vi "Lab Panel V6.00.vi"() -> ()   [LabVIEW 2017] (continued)
                n2898 = Index Array(array=w5298, index=4) -> (element=w5301:bool)
                n2899 = Not(x=w5301) -> (.not. x?=w5299:bool)
                n2900 = And(x=w5299, y=w5297) -> (x .and. y?=w5296:bool)
                n2901 = case shown="True" w5296 {
                  tunnel: w5304 -> [_ w5318]
                  tunnel: w5302 -> [_ w5315]
                  tunnel: w5303 -> [_ w5314]
                  frame False {
                  }
                  frame True {
                    n2902 = local read "TEMP START LAB05-2"() -> (w5320:cluster{"TL":dbl, "TN":dbl})
                    n2903 = local read "FAIL LAB05-2"() -> (w5311:cluster{"LO":dbl, "HI":dbl})
                    n2904 = local read "TDMS LAB05-2"() -> (w5319:refnum<k34>)
                    n2905 = local read "SET LAB05-2"() -> (w5316:T5)
                    n2906 = local read "DISP LAB05-2"() -> (w5317:T4)
                    n2907 = local read "SIG LAB05-2"() -> (w5321:T2)
                    n2908 = local read "RESULT LAB05-2"() -> (w5308:bool)
                    n2909 = Bundle("FAIL LAB05-2"=w5311, "SIG LAB05-2"=w5321, "TEMP START LAB05-2"=w5320, "DISP LAB05-2"=w5317, "SET LAB05-2"=w5316, "TDMS LAB05-2"=w5319) -> (w5306:T46)  [unwired: 1 in]
                    n2910 = call "sub vi - cycle&temp fail v7.vi"("Amps Lo?"=w5318, "Input Cluster"=w5306, "SELECT"=w5315, "Amps Hi?"=w5314, "Result In"=w5308, "Panel"=u64 10) -> ("(FAIL) out"=w5310:cluster{"FAIL LO":dbl, "FAIL HI":dbl}, "(DISP) out"=w5313:T4, "T-RISE"=w5307:cluster{"T-RISE (L)":dbl, "T-RISE (N)":dbl}, "Result Out"=w5309:bool, "file error"=w5312:errorcluster)  [unwired: 9 in]
                    n2911 = local write "TEMP RISE LAB05-2"(w5307) -> ()
                    n2912 = local write "FAIL LAB05-2"(w5310) -> ()
                    n2913 = local write "DISP LAB05-2"(w5313) -> ()
                    n2914 = local write "RESULT LAB05-2"(w5309) -> ()
                    n2915 = local write "data file error"(w5312) -> ()
                  }
                }
              }
            }
            n2916 = global write "Global 1.vi" "fail count"(w5035) -> ()
          }
          frame #17 {
            # "run calibration routine"
            n2917 = local read "SET (cal)"() -> (w5322:bool)
            n2918 = case shown="True" w5322 {
              frame False {
              }
              frame True {
                n2919 = stacked-sequence {
                  seq-local: [w5323 _ _] -> [_ w5325 _]
                  frame #0 {
                    n2920 = call "CALIBRATION PASSWORD"() -> ("PASSWORD"=w5323:string)  [unwired: 17 in, 2 out]
                  }
                  frame #1 {
                    n2921 = Equal?(x=w5325, y="7777") -> (x = y?=w5324:bool)
                    n2922 = case shown="True" w5324 {
                      frame False {
                      }
                      frame True {
                        n2923 = stacked-sequence {
                          frame #0 {
                            n2924 = local read "SAMPLES"() -> (w5327:dbl)
                            n2925 = local read "AI Task2"() -> (w5328:u32)
                            n2926 = local read "AI Task1"() -> (w5329:u32)
                            n2927 = local read "AI Task0"() -> (w5330:u64)
                            n2928 = local read "Temp Test Cal"() -> (w5331:dbl)
                            n2929 = call "sub vi - calibration v2.vi"("Samples"=w5327, "Task2"=w5328, "Task1"=w5329, "Task0"=w5330, "Temp Test Cal"=w5331) -> ()  [unwired: 7 in]
                          }
                          frame #1 {
                            n2930 = call "sub vi - get calibration values v1.vi"() -> ("TEMP REF CAL"=w5332:dbl, "LAB01 (CAL)"=w5337:T15, "LAB02 (CAL)"=w5336:T16, "LAB03 (CAL)"=w5335:T15, "LAB04 (CAL)"=w5334:T15, "calibration file error out"=w5338:errorcluster, "LAB05 (CAL)"=w5333:T15)  [unwired: 9 in]
                            n2931 = local write "TEMP REF cal"(w5332) -> ()
                            n2932 = local write "cal file error out"(w5338) -> ()
                            n2933 = local write "CAL LAB04"(w5334) -> ()
                            n2934 = local write "CAL LAB05"(w5333) -> ()
                            n2935 = local write "CAL LAB01"(w5337) -> ()
                            n2936 = local write "CAL LAB02"(w5336) -> ()
                            n2937 = local write "CAL LAB03"(w5335) -> ()
                          }
                        }
                      }
                    }
                  }
                  frame #2 {
                    n2938 = local write "SET (cal)"(FALSE) -> ()
                  }
                }
              }
            }
          }
          frame #18 {
            # "save certain settings to file"
            n2939 = String To Path(string="c:\\crabtree\\Set Up\\") -> (path=w5341:path)
            n2940 = Build Path(base path=w5341, name or relative path="settings.bin") -> (appended path=w5343:path)
            n2941 = Build Path(base path=w5341, name or relative path="mail.bin") -> (appended path=w5340:path)
            n2942 = Create Folder(path (use dialog)=w5341) -> (error out=w5346:errorcluster)  [unwired: 2 in, 2 out]
            n2943 = call <vilib>:"Clear Errors.vi"("error in (no error)"=w5346) -> ()  [unwired: 5 in, 2 out]
            n2944 = stacked-sequence {
              seq-local: [w5358 _] -> [_ w5371]
              tunnel: w5343 -> [_ w5372]
              tunnel: w5340 -> [_ w5370]
              frame #0 {
                n2945 = local read "C drive data root dir"() -> (w5357:path)
                n2946 = local read "Select COM port"() -> (w5354:refnum<visa-resource-name>)
                n2947 = local read "Network Directory"() -> (w5363:path)
                n2948 = local read "SET LAB05-2"() -> (w5362:T5)
                n2949 = local read "SET LAB05-1"() -> (w5361:T5)
                n2950 = local read "SET LAB04-2"() -> (w5360:T5)
                n2951 = local read "SET LAB03-2"() -> (w5364:T5)
                n2952 = local read "SET LAB04-1"() -> (w5359:T5)
                n2953 = local read "SET LAB03-1"() -> (w5365:T5)
                n2954 = local read "SET LAB02-2"() -> (w5366:T5)
                n2955 = local read "SET LAB02-1"() -> (w5367:T5)
                n2956 = local read "SET LAB01-2"() -> (w5368:T5)
                n2957 = local read "SET LAB01-1"() -> (w5369:T6)
                n2958 = local read "Temp Delay Lps"() -> (w5353:dbl)
                n2959 = local read "Amps Fail level"() -> (w5349:dbl)
                n2960 = local read "Temp Test Cal"() -> (w5350:dbl)
                n2961 = local read "Temp Value"() -> (w5352:dbl)
                n2962 = local read "Mail Test File To:"() -> (w5348:string)
                n2963 = local read "Fail Loops"() -> (w5351:dbl)
                n2964 = local read "Mail Test Fail"() -> (w5347:bool)
                n2965 = local read "RATE (Hz)"() -> (w5356:dbl)
                n2966 = local read "SAMPLES"() -> (w5355:dbl)
                n2967 = Bundle("SET LAB01-1"=w5369, "SET LAB01-2"=w5368, "SET LAB02-1"=w5367, "SET LAB02-2"=w5366, "SET LAB03-1"=w5365, "SET LAB03-2"=w5364, "SET LAB04-1"=w5359, "SET LAB04-2"=w5360, "SET LAB05-1"=w5361, "SET LAB05-2"=w5362, "Network Directory"=w5363, "C drive data root dir"=w5357, "RATE (Hz)"=w5356, "SAMPLES"=w5355, "Select COM port"=w5354, "Temp Delay Lps"=w5353, "Temp Value"=w5352, "Fail Loops"=w5351, "Temp Test Cal"=w5350, "Amps Fail level"=w5349, "Mail Test File To:"=w5348, "Mail Test Fail"=w5347) -> (w5358:T25)  [unwired: 1 in]
              }
              frame #1 {
                n2968 = event shown="[1] \"SET LAB01-1\", \"SET LAB01-2\", \"SET LAB02-1\", \"SET LAB02-2\", \"SET LAB03-1\", \"SET LAB03-2\", \"SET LAB04-1\", \"SET LAB04-2\", \"SET LAB05-1\", \"SET LAB05-2\", \"Network Directory\", \"C drive data root dir\", \"RATE (Hz)\", \"SAMPLES\", \"Select COM port\", \"Temp Delay Lps\", \"Temp Value\", \"Fail Loops\", \"Temp Test Cal\", \"Amps Fail level\", \"Mail Test File To:\", \"Mail Test Fail\": Value Change" {
                  selector: _ -> [_ _ _]
                  dyn-events: _ -> [_ _ _]
                  timeout: 10.0 -> [_ _ _]
                  tunnel: w5372 -> [_ w5374 _]
                  tunnel: w5371 -> [_ w5375 _]
                  tunnel: w5370 -> [_ _ w5386]
                  event Timeout {
                    n2969 = event-data() -> ()  [unwired: 1 in, 3 out]
                  }
                  event "SET LAB01-2", "SET LAB02-1", "SET LAB02-2", "SET LAB03-1", "SET LAB03-2", "SET LAB04-1", "SET LAB04-2", "SET LAB05-1", "SET LAB05-2", "Network Directory", "C drive data root dir", "RATE (Hz)", "SAMPLES", "Select COM port", "Temp Delay Lps", "Temp Value", "Fail Loops", "Temp Test Cal", "Amps Fail level", "Mail Test File To:", "Mail Test Fail": Value Change {
                    n2970 = event-data() -> ()  [unwired: 1 in, 6 out]
                    n2971 = Open/Create/Replace File(file path (use dialog)=w5374, operation (0:open)=T18."replace or create") -> (refnum out=w5380:refnum<file>, error out=w5379:errorcluster)  [unwired: 4 in, 1 out]
                    n2972 = Write to Binary File(file (use dialog)=w5380, data=w5375, error in=w5379) -> (refnum out=w5378:refnum<file>, error out=w5377:errorcluster)  [unwired: 3 in, 1 out]
                    n2973 = Close File(refnum=w5378, error in=w5377) -> (error out=w5376:errorcluster)  [unwired: 1 out]
                    n2974 = local write "data file error"(w5376) -> ()
                  }
                  event "MAIL SETTINGS.OUT SERVER ADDRESS", "MAIL SETTINGS.FROM ACCOUNT", "MAIL SETTINGS.USER NAME", "MAIL SETTINGS.PASSWORD", "Auto Mail Send", "TO (string):": Value Change {
                    n2975 = event-data() -> ()  [unwired: 1 in, 6 out]
                    n2976 = local read "Auto Mail Send"() -> (w5383:bool)
                    n2977 = local read "MAIL SETTINGS"() -> (w5385:T8)
                    n2978 = local read "TO (string):"() -> (w5382:string)
                    n2979 = Open/Create/Replace File(file path (use dialog)=w5386, operation (0:open)=T18."replace or create") -> (refnum out=w5391:refnum<file>, error out=w5390:errorcluster)  [unwired: 4 in, 1 out]
                    n2980 = Bundle("MAIL SETTINGS"=w5385, "Auto Mail Send"=w5383, "TO (string):"=w5382) -> (w5384:T47)  [unwired: 1 in]
                    n2981 = Write to Binary File(file (use dialog)=w5391, data=w5384, error in=w5390) -> (refnum out=w5389:refnum<file>, error out=w5388:errorcluster)  [unwired: 3 in, 1 out]
                    n2982 = Close File(refnum=w5389, error in=w5388) -> (error out=w5387:errorcluster)  [unwired: 1 out]
                    n2983 = local write "data file error"(w5387) -> ()
                  }
                }
              }
            }
          }
          frame #19 {
            # "mail control"
            n2984 = local read "MAIL SETTINGS"() -> (w5408:T8)
            n2985 = local read "Auto Mail Send"() -> (w5394:bool)
            n2986 = Unbundle By Name(w5408) -> ("OUT SERVER ADDRESS"=w5407:string, "FROM ACCOUNT"=w5406:string, "TEST MAIL"=w5405:bool)
            n2987 = stacked-sequence {
              tunnel: "TO (string):" -> [_ w5447]
              tunnel: w5408 -> [w5413 w5446]
              tunnel: w5407 -> [w5412 w5445]
              tunnel: w5406 -> [w5411 w5444]
              tunnel: w5405 -> [w5410 _]
              tunnel: w5394 -> [_ w5443]
              tunnel: w5404 -> [_ w5442]
              tunnel: w5403 -> [_ w5441]
              tunnel: w5402 -> [_ w5440]
              tunnel: w5401 -> [_ w5439]
              tunnel: w5400 -> [_ w5438]
              tunnel: w5399 -> [_ w5437]
              tunnel: w5398 -> [_ w5436]
              tunnel: w5397 -> [_ w5435]
              tunnel: w5396 -> [_ w5434]
              tunnel: w5395 -> [_ w5433]
              tunnel: "TO (string):" -> [w5409 _]
              frame #0 {
                # "mail test"
                n2988 = case shown="True" w5410 {
                  tunnel: w5413 -> [_ w5417]
                  tunnel: w5409 -> [_ w5416]
                  tunnel: w5412 -> [_ w5415]
                  tunnel: w5411 -> [_ w5414]
                  frame False {
                  }
                  frame True {
                    n2989 = stacked-sequence {
                      seq-local: [_ _ w5427 _] -> [_ _ _ w5428]
                      tunnel: w5417 -> [w5420 _ _ w5432]
                      tunnel: w5416 -> [_ _ w5425 _]
                      tunnel: w5415 -> [_ _ w5423 _]
                      tunnel: w5414 -> [_ _ w5424 _]
                      frame #0 {
                        n2990 = Bundle(cluster=w5420, "TEST MAIL STATUS"="TEST START") -> (w5418:T8)  [unwired: 6 in]
                        n2991 = local write "MAIL SETTINGS"(w5418) -> ()
                      }
                      frame #1 {
                        n2992 = Wait (ms)(milliseconds to wait=500) -> ()  [unwired: 1 out]
                      }
                      frame #2 {
                        n2993 = call "Lab Send Mail Test.vi"("TO:"=w5425, "subject"="MAIL TEST FROM LAB PANEL", "from"=w5424, "out going server"=w5423, "message"="TEST MESSAGE") -> ("error out"=w5427:errorcluster)  [unwired: 10 in]
                      }
                      frame #3 {
                        n2994 = Bundle(cluster=w5432, "TEST MAIL"=FALSE, "TEST MAIL STATUS"="TEST END", "mail error"=w5428) -> (w5430:T8)  [unwired: 4 in]
                        n2995 = local write "MAIL SETTINGS"(w5430) -> ()
                      }
                    }
                  }
                }
              }
              frame #1 {
                # "mail report"
                n2996 = stacked-sequence {
                  seq-local: [_ w5490 _ _] -> [_ _ _ w5680]
                  seq-local: [_ _ w5593 _] -> [_ _ _ w5670]
                  seq-local: [w5457 _ _ _] -> [_ w5507 _ _]
                  seq-local: [w5456 _ _ _] -> [_ w5506 _ _]
                  seq-local: [w5454 _ _ _] -> [_ w5504 _ _]
                  seq-local: [w5455 _ _ _] -> [_ w5505 _ _]
                  seq-local: [w5453 _ _ _] -> [_ w5503 _ _]
                  seq-local: [w5452 _ _ _] -> [_ w5498 _ _]
                  seq-local: [w5451 _ _ _] -> [_ w5499 _ _]
                  seq-local: [w5450 _ _ _] -> [_ w5500 _ _]
                  seq-local: [w5449 _ _ _] -> [_ w5501 _ _]
                  seq-local: [w5448 _ _ _] -> [_ w5502 _ _]
                  tunnel: w5447 -> [_ _ _ w5681]
                  tunnel: w5446 -> [_ _ _ w5664]
                  tunnel: w5445 -> [_ _ _ w5678]
                  tunnel: w5444 -> [_ _ _ w5677]
                  tunnel: w5443 -> [w5488 _ _ w5672]
                  tunnel: w5442 -> [_ _ w5623 _]
                  tunnel: w5441 -> [_ _ w5620 _]
                  tunnel: w5440 -> [_ _ w5619 _]
                  tunnel: w5439 -> [_ _ w5618 _]
                  tunnel: w5438 -> [_ _ w5617 _]
                  tunnel: w5437 -> [_ _ w5616 _]
                  tunnel: w5436 -> [_ _ w5615 _]
                  tunnel: w5435 -> [_ _ w5614 _]
                  tunnel: w5434 -> [_ _ w5613 _]
                  tunnel: w5433 -> [_ _ w5612 _]
                  frame #0 {
                    n2997 = case shown="False" w5488 {
                      frame False {
                        n2998 = local write "mail control"("") -> ()
                      }
                      frame True {
                      }
                    }
                    n2999 = local read "SET LAB01-1"() -> (w5487:T6)
                    n3000 = local read "SET LAB01-2"() -> (w5486:T5)
                    n3001 = local read "SET LAB02-1"() -> (w5485:T5)
                    n3002 = local read "SET LAB02-2"() -> (w5484:T5)
                    n3003 = local read "SET LAB03-1"() -> (w5483:T5)
                    n3004 = local read "SET LAB04-1"() -> (w5481:T5)
                    n3005 = local read "SET LAB05-1"() -> (w5479:T5)
                    n3006 = local read "SET LAB03-2"() -> (w5482:T5)
                    n3007 = local read "SET LAB04-2"() -> (w5480:T5)
                    n3008 = local read "SET LAB05-2"() -> (w5478:T5)
                    n3009 = Unbundle(w5483) -> ("DESCRIPTION"=w5463:string)  [unwired: 4 out]
                    n3010 = Unbundle(w5482) -> ("DESCRIPTION"=w5462:string)  [unwired: 4 out]
                    n3011 = Unbundle(w5481) -> ("DESCRIPTION"=w5461:string)  [unwired: 4 out]
                    n3012 = Unbundle(w5478) -> ("DESCRIPTION"=w5458:string)  [unwired: 4 out]
                    n3013 = Unbundle(w5484) -> ("DESCRIPTION"=w5464:string)  [unwired: 4 out]
                    n3014 = Unbundle(w5480) -> ("DESCRIPTION"=w5460:string)  [unwired: 4 out]
                    n3015 = Unbundle(w5487) -> ("DESCRIPTION"=w5476:string)  [unwired: 4 out]
                    n3016 = Unbundle(w5485) -> ("DESCRIPTION"=w5465:string)  [unwired: 4 out]
                    n3017 = Unbundle(w5479) -> ("DESCRIPTION"=w5459:string)  [unwired: 4 out]
                    n3018 = Unbundle(w5486) -> ("DESCRIPTION"=w5466:string)  [unwired: 4 out]
                    n3019 = Concatenate Strings("[LAB05-2/", w5458) -> (w5448:string)
                    n3020 = Concatenate Strings("[LAB05-1/", w5459) -> (w5449:string)
                    n3021 = Concatenate Strings("[LAB04-2/", w5460) -> (w5450:string)
                    n3022 = Concatenate Strings("[LAB03-2/", w5462) -> (w5452:string)
                    n3023 = Concatenate Strings("[LAB04-1/", w5461) -> (w5451:string)
                    n3024 = Concatenate Strings("[LAB03-1/", w5463) -> (w5453:string)
                    n3025 = Concatenate Strings("[LAB01-2/", w5466) -> (w5456:string)
                    n3026 = Concatenate Strings("[LAB02-2/", w5464) -> (w5454:string)
                    n3027 = Concatenate Strings("[LAB01-1/", w5476) -> (w5457:string)
                    n3028 = Concatenate Strings("[LAB02-1/", w5465) -> (w5455:string)
                  }
                  frame #1 {
                    w5511 = "/"
                    w5512 = 2.0
                    n3029 = local read "DISP LAB01-1"() -> (w5592:T4)
                    n3030 = local read "DISP LAB01-2"() -> (w5591:T4)
                    n3031 = local read "DISP LAB02-1"() -> (w5590:T4)
                    n3032 = local read "DISP LAB03-2"() -> (w5587:T4)
                    n3033 = local read "DISP LAB02-2"() -> (w5589:T4)
                    n3034 = local read "DISP LAB03-1"() -> (w5588:T4)
                    n3035 = local read "DISP LAB04-2"() -> (w5585:T4)
                    n3036 = local read "DISP LAB04-1"() -> (w5586:T4)
                    n3037 = local read "DISP LAB05-1"() -> (w5584:T4)
                    n3038 = local read "DISP LAB05-2"() -> (w5583:T4)
                    n3039 = Unbundle By Name(w5592) -> ("CYCLE"=w5580:dbl, "MINS"=w5579:dbl, "STATUS"=w5576:string)
                    n3040 = Unbundle(w5591) -> ("CYCLE"=w5575:dbl, "MINS"=w5574:dbl, "STATUS"=w5571:string)
                    n3041 = Unbundle(w5590) -> ("CYCLE"=w5568:dbl, "MINS"=w5567:dbl, "STATUS"=w5566:string)
                    n3042 = Unbundle(w5587) -> ("CYCLE"=w5555:dbl, "MINS"=w5554:dbl, "STATUS"=w5551:string)
                    n3043 = Unbundle(w5588) -> ("CYCLE"=w5560:dbl, "MINS"=w5559:dbl, "STATUS"=w5556:string)
                    n3044 = Unbundle(w5589) -> ("CYCLE"=w5565:dbl, "MINS"=w5564:dbl, "STATUS"=w5561:string)
                    n3045 = Unbundle(w5586) -> ("CYCLE"=w5550:dbl, "MINS"=w5549:dbl, "STATUS"=w5546:string)
                    n3046 = Unbundle(w5585) -> ("CYCLE"=w5545:dbl, "MINS"=w5544:dbl, "STATUS"=w5541:string)
                    n3047 = Unbundle(w5584) -> ("CYCLE"=w5540:dbl, "MINS"=w5539:dbl, "STATUS"=w5536:string)
                    n3048 = Unbundle(w5583) -> ("CYCLE"=w5582:dbl, "MINS"=w5581:dbl, "STATUS"=w5533:string)
                    n3049 = Number To Decimal String(number=w5568) -> (decimal integer string=w5570:string)  [unwired: 1 in]
                    n3050 = Number To Decimal String(number=w5565) -> (decimal integer string=w5563:string)  [unwired: 1 in]
                    n3051 = Number To Decimal String(number=w5560) -> (decimal integer string=w5558:string)  [unwired: 1 in]
                    n3052 = Number To Decimal String(number=w5575) -> (decimal integer string=w5573:string)  [unwired: 1 in]
                    n3053 = Number To Decimal String(number=w5555) -> (decimal integer string=w5553:string)  [unwired: 1 in]
                    n3054 = Number To Decimal String(number=w5580) -> (decimal integer string=w5578:string)  [unwired: 1 in]
                    n3055 = Number To Decimal String(number=w5582) -> (decimal integer string=w5535:string)  [unwired: 1 in]
                    n3056 = Number To Decimal String(number=w5550) -> (decimal integer string=w5548:string)  [unwired: 1 in]
                    n3057 = Number To Decimal String(number=w5545) -> (decimal integer string=w5543:string)  [unwired: 1 in]
                    n3058 = Number To Decimal String(number=w5540) -> (decimal integer string=w5538:string)  [unwired: 1 in]
                    n3059 = Number To Fractional String(number=w5567, precision (6)=w5512) -> (F-format string=w5569:string)  [unwired: 2 in]
                    n3060 = Number To Fractional String(number=w5554, precision (6)=w5512) -> (F-format string=w5552:string)  [unwired: 2 in]
                    n3061 = Number To Fractional String(number=w5564, precision (6)=w5512) -> (F-format string=w5562:string)  [unwired: 2 in]
                    n3062 = Number To Fractional String(number=w5559, precision (6)=w5512) -> (F-format string=w5557:string)  [unwired: 2 in]
                    n3063 = Number To Fractional String(number=w5544, precision (6)=w5512) -> (F-format string=w5542:string)  [unwired: 2 in]
                    n3064 = Number To Fractional String(number=w5549, precision (6)=w5512) -> (F-format string=w5547:string)  [unwired: 2 in]
                    n3065 = Number To Fractional String(number=w5574, precision (6)=w5512) -> (F-format string=w5572:string)  [unwired: 2 in]
                    n3066 = Number To Fractional String(number=w5539, precision (6)=w5512) -> (F-format string=w5537:string)  [unwired: 2 in]
                    n3067 = Number To Fractional String(number=w5579, precision (6)=w5512) -> (F-format string=w5577:string)  [unwired: 2 in]
                    n3068 = Number To Fractional String(number=w5581, precision (6)=w5512) -> (F-format string=w5534:string)  [unwired: 2 in]
                    n3069 = Concatenate Strings(w5511, w5553, w5511, w5552, w5511, w5551) -> (w5527:string)
                    n3070 = Concatenate Strings(w5511, w5548, w5511, w5547, w5511, w5546) -> (w5526:string)
                    n3071 = Concatenate Strings(w5511, w5543, w5511, w5542, w5511, w5541) -> (w5525:string)
                    n3072 = Concatenate Strings(w5511, w5538, w5511, w5537, w5511, w5536) -> (w5524:string)
                    n3073 = Concatenate Strings(w5511, w5535, w5511, w5534, w5511, w5533) -> (w5523:string)
                    n3074 = Concatenate Strings(w5511, w5578, w5511, w5577, w5511, w5576) -> (w5532:string)
                    n3075 = Concatenate Strings(w5511, w5558, w5511, w5557, w5511, w5556) -> (w5528:string)
                    n3076 = Concatenate Strings(w5511, w5573, w5511, w5572, w5511, w5571) -> (w5531:string)
                    n3077 = Concatenate Strings(w5511, w5570, w5511, w5569, w5511, w5566) -> (w5530:string)
                    n3078 = Concatenate Strings(w5511, w5563, w5511, w5562, w5511, w5561) -> (w5529:string)
                    n3079 = Concatenate Strings("]", "\r") -> (w5508:string)
                    n3080 = Concatenate Strings(w5503, w5528, w5508) -> (w5518:string)
                    n3081 = Concatenate Strings(w5505, w5530, w5508) -> (w5520:string)
                    n3082 = Concatenate Strings(w5504, w5529, w5508) -> (w5519:string)
                    n3083 = Concatenate Strings(w5500, w5525, w5508) -> (w5515:string)
                    n3084 = Concatenate Strings(w5501, w5524, w5508) -> (w5516:string)
                    n3085 = Concatenate Strings(w5499, w5526, w5508) -> (w5514:string)
                    n3086 = Concatenate Strings(w5498, w5527, w5508) -> (w5513:string)
                    n3087 = Concatenate Strings(w5502, w5523, w5508) -> (w5517:string)
                    n3088 = Concatenate Strings(w5506, w5531, w5508) -> (w5521:string)
                    n3089 = Concatenate Strings(w5507, w5532, w5508) -> (w5522:string)
                    n3090 = Concatenate Strings(w5522, w5521, w5520, w5519, w5518, w5513, w5514, w5515, w5516, w5517) -> (w5491:string)
                    n3091 = Concatenate Strings("[PANEL/", "DESC/", "CYCLES/", "MINS/", "STATUS]", "\r", w5491) -> (w5490:string)
                    "MAIL REPORT" <- w5490
                    n3092 = global write "Global display 3.vi" "log all"(w5490) -> ()
                  }
                  frame #2 {
                    w5621 = "END"
                    n3093 = local read "mail control"() -> (w5622:string)
                    n3094 = case shown="False" w5617 {
                      tunnel: w5622 -> [w5646 _]
                      tunnel: w5621 -> [w5645 _]
                      tunnel: [w5644 FALSE] -> w5607
                      frame False {
                        n3095 = Equal?(x=w5646, y=w5645) -> (x = y?=w5644:bool)
                      }
                      frame True {
                      }
                    }
                    n3096 = case shown="False" w5623 {
                      tunnel: w5622 -> [w5662 _]
                      tunnel: w5621 -> [w5661 _]
                      tunnel: [w5660 FALSE] -> w5611
                      frame False {
                        n3097 = Equal?(x=w5662, y=w5661) -> (x = y?=w5660:bool)
                      }
                      frame True {
                      }
                    }
                    n3098 = case shown="False" w5620 {
                      tunnel: w5622 -> [w5658 _]
                      tunnel: w5621 -> [w5657 _]
                      tunnel: [w5656 FALSE] -> w5610
                      frame False {
                        n3099 = Equal?(x=w5658, y=w5657) -> (x = y?=w5656:bool)
                      }
                      frame True {
                      }
                    }
                    n3100 = case shown="False" w5618 {
                      tunnel: w5622 -> [w5650 _]
                      tunnel: w5621 -> [w5649 _]
                      tunnel: [w5648 FALSE] -> w5608
                      frame False {
                        n3101 = Equal?(x=w5650, y=w5649) -> (x = y?=w5648:bool)
                      }
                      frame True {
                      }
                    }
                    n3102 = case shown="False" w5619 {
                      tunnel: w5622 -> [w5654 _]
                      tunnel: w5621 -> [w5653 _]
                      tunnel: [w5652 FALSE] -> w5609
                      frame False {
                        n3103 = Equal?(x=w5654, y=w5653) -> (x = y?=w5652:bool)
                      }
                      frame True {
                      }
                    }
                    n3104 = Or(x=w5609, y=w5608) -> (x .or. y?=w5600:bool)
                    n3105 = Or(x=w5611, y=w5610) -> (x .or. y?=w5601:bool)
                    n3106 = Or(x=w5601, y=w5600) -> (x .or. y?=w5596:bool)
                    n3107 = case shown="False" w5613 {
                      tunnel: w5622 -> [w5630 _]
                      tunnel: w5621 -> [w5629 _]
                      tunnel: [w5628 FALSE] -> w5602
                      frame False {
                        n3108 = Equal?(x=w5630, y=w5629) -> (x = y?=w5628:bool)
                      }
                      frame True {
                      }
                    }
                    n3109 = case shown="False" w5612 {
                      tunnel: w5622 -> [w5626 _]
                      tunnel: w5621 -> [w5625 _]
                      tunnel: [w5624 FALSE] -> w5606
                      frame False {
                        n3110 = Equal?(x=w5626, y=w5625) -> (x = y?=w5624:bool)
                      }
                      frame True {
                      }
                    }
                    n3111 = case shown="False" w5614 {
                      tunnel: w5622 -> [w5634 _]
                      tunnel: w5621 -> [w5633 _]
                      tunnel: [w5632 FALSE] -> w5603
                      frame False {
                        n3112 = Equal?(x=w5634, y=w5633) -> (x = y?=w5632:bool)
                      }
                      frame True {
                      }
                    }
                    n3113 = case shown="False" w5616 {
                      tunnel: w5622 -> [w5642 _]
                      tunnel: w5621 -> [w5641 _]
                      tunnel: [w5640 FALSE] -> w5605
                      frame False {
                        n3114 = Equal?(x=w5642, y=w5641) -> (x = y?=w5640:bool)
                      }
                      frame True {
                      }
                    }
                    n3115 = case shown="False" w5615 {
                      tunnel: w5622 -> [w5638 _]
                      tunnel: w5621 -> [w5637 _]
                      tunnel: [w5636 FALSE] -> w5604
                      frame False {
                        n3116 = Equal?(x=w5638, y=w5637) -> (x = y?=w5636:bool)
                      }
                      frame True {
                      }
                    }
                    n3117 = Or(x=w5605, y=w5604) -> (x .or. y?=w5599:bool)
                    n3118 = Or(x=w5603, y=w5602) -> (x .or. y?=w5598:bool)
                    n3119 = Or(x=w5606, y=w5607) -> (x .or. y?=w5594:bool)
                    n3120 = Or(x=w5599, y=w5598) -> (x .or. y?=w5597:bool)
                    n3121 = Or(x=w5596, y=w5597) -> (x .or. y?=w5595:bool)
                    n3122 = Or(x=w5595, y=w5594) -> (x .or. y?=w5593:bool)
                  }
                  frame #3 {
                    n3123 = local read "on loops"() -> (w5676:dbl)
                    n3124 = local read "jig cycle"() -> (w5673:dbl)
                    n3125 = local read "Send Mail Now"() -> (w5667:bool)
                    n3126 = Add(x=w5676, y=5.0) -> (x+y=w5674:dbl)
                    n3127 = Equal?(x=w5673, y=w5674) -> (x = y?=w5668:bool)
                    n3128 = And(x=w5668, y=w5667) -> (x .and. y?=w5666:bool)
                    n3129 = And(x=w5672, y=w5668) -> (x .and. y?=w5671:bool)
                    n3130 = And(x=w5671, y=w5670) -> (x .and. y?=w5669:bool)
                    n3131 = Or(x=w5669, y=w5666) -> (x .or. y?=w5665:bool)
                    n3132 = case shown="True" w5665 {
                      tunnel: w5681 -> [_ w5687]
                      tunnel: w5680 -> [_ w5686]
                      tunnel: "Lab Panel Test Status" -> [_ w5685]
                      tunnel: w5678 -> [_ w5684]
                      tunnel: w5677 -> [_ w5683]
                      tunnel: w5664 -> [_ w5682]
                      frame False {
                      }
                      frame True {
                        n3133 = stacked-sequence {
                          tunnel: w5687 -> [w5696 _]
                          tunnel: w5686 -> [w5695 _]
                          tunnel: w5685 -> [w5694 _]
                          tunnel: w5684 -> [w5693 _]
                          tunnel: w5683 -> [w5692 _]
                          tunnel: w5682 -> [w5691 _]
                          frame #0 {
                            n3134 = call "Lab Send Mail Test.vi"("TO:"=w5696, "subject"=w5694, "Info"="Test station status report", "from"=w5692, "out going server"=w5693, "message"=w5695) -> ("error out"=w5690:errorcluster)  [unwired: 9 in]
                            n3135 = Bundle(cluster=w5691, "mail error"=w5690) -> (w5689:T8)  [unwired: 6 in]
                            n3136 = local write "MAIL SETTINGS"(w5689) -> ()
                          }
                          frame #1 {
                            n3137 = local write "mail control"("") -> ()
                            n3138 = local write "Send Mail Now"(FALSE) -> ()
                          }
                        }
                      }
                    }
                  }
                }
              }
            }
          }
          frame #20 {
            # "save jig cycle values once all run switches are off"
            n3139 = stacked-sequence {
              tunnel: w5708 -> [_ w5737]
              tunnel: w5707 -> [_ w5736]
              tunnel: w5706 -> [_ w5735]
              tunnel: w5705 -> [_ w5734]
              tunnel: w5704 -> [_ w5733]
              tunnel: w5703 -> [_ w5732]
              tunnel: w5702 -> [_ w5731]
              tunnel: w5701 -> [_ w5730]
              tunnel: w5700 -> [_ w5729]
              tunnel: w5699 -> [_ w5728]
              frame #0 {
              }
              frame #1 {
                n3140 = Not(x=w5728) -> (.not. x?=w5711:bool)
                n3141 = Not(x=w5736) -> (.not. x?=w5726:bool)
                n3142 = Not(x=w5733) -> (.not. x?=w5721:bool)
                n3143 = Not(x=w5731) -> (.not. x?=w5717:bool)
                n3144 = Not(x=w5729) -> (.not. x?=w5713:bool)
                n3145 = Not(x=w5737) -> (.not. x?=w5727:bool)
                n3146 = Not(x=w5735) -> (.not. x?=w5725:bool)
                n3147 = Not(x=w5732) -> (.not. x?=w5719:bool)
                n3148 = Not(x=w5734) -> (.not. x?=w5723:bool)
                n3149 = Not(x=w5730) -> (.not. x?=w5715:bool)
                n3150 = local read "Save JC"() -> (w5739:bool)
                n3151 = And(x=w5727, y=w5726) -> (x .and. y?=w5724:bool)
                n3152 = And(x=w5724, y=w5725) -> (x .and. y?=w5722:bool)
                n3153 = And(x=w5722, y=w5723) -> (x .and. y?=w5720:bool)
                n3154 = And(x=w5720, y=w5721) -> (x .and. y?=w5718:bool)
                n3155 = And(x=w5718, y=w5719) -> (x .and. y?=w5716:bool)
                n3156 = And(x=w5716, y=w5717) -> (x .and. y?=w5714:bool)
                n3157 = And(x=w5714, y=w5715) -> (x .and. y?=w5712:bool)
                n3158 = And(x=w5712, y=w5713) -> (x .and. y?=w5710:bool)
                n3159 = And(x=w5710, y=w5711) -> (x .and. y?=w5709:bool)
                n3160 = And(x=w5709, y=w5739) -> (x .and. y?=w5738:bool)
                n3161 = case shown="True" w5738 {
                  tunnel: w5709 -> [w5740 _]
                  frame False {
                    n3162 = case shown="False" w5740 {
                      frame False {
                        n3163 = local write "Save JC"(TRUE) -> ()
                      }
                      frame True {
                      }
                    }
                  }
                  frame True {
                    n3164 = stacked-sequence {
                      frame #0 {
                        n3165 = String To Path(string="c:\\crabtree\\Jig Cycles\\") -> (path=w5752:path)
                        n3166 = Build Path(base path=w5752, name or relative path="jigcycles.bin") -> (appended path=w5750:path)
                        n3167 = Create Folder(path (use dialog)=w5752) -> (error out=w5754:errorcluster)  [unwired: 2 in, 2 out]
                        n3168 = local read "JIG RELAY CYCLES"() -> (w5744:T9)
                        n3169 = call <vilib>:"Clear Errors.vi"("error in (no error)"=w5754) -> ()  [unwired: 5 in, 2 out]
                        n3170 = local write "Save JC"(FALSE) -> ()
                        n3171 = Open/Create/Replace File(file path (use dialog)=w5750, operation (0:open)=T18."replace or create") -> (refnum out=w5748:refnum<file>, error out=w5749:errorcluster)  [unwired: 4 in, 1 out]
                        n3172 = Write to Binary File(file (use dialog)=w5748, data=w5744, error in=w5749) -> (refnum out=w5747:refnum<file>, error out=w5746:errorcluster)  [unwired: 3 in, 1 out]
                        n3173 = Close File(refnum=w5747, error in=w5746) -> (error out=w5745:errorcluster)  [unwired: 1 out]
                        n3174 = local write "data file error"(w5745) -> ()
                      }
                      frame #1 {
                        n3175 = local read "JIG RELAY CYCLES"() -> (w5777:T9)
                        n3176 = Unbundle By Name(w5777) -> ("LAB01-1"=w5772:dbl, "LAB01-2"=w5771:dbl, "LAB02-1"=w5769:dbl, "LAB02-2"=w5768:dbl, "LAB03-1"=w5766:dbl, "LAB03-2"=w5763:dbl, "LAB04-1"=w5762:dbl, "LAB04-2"=w5760:dbl, "LAB05-1"=w5758:dbl, "LAB05-2"=w5756:dbl)
                        n3177 = stacked-sequence {
                          tunnel: w5772 -> [w5780 _ _ _ _ _ _ _ _ _]
                          tunnel: 1000000 -> [w5783 w5793 w5803 w5813 w5823 w5833 w5843 w5853 w5863 w5873]
                          tunnel: [w5781 _ _ _ _ _ _ _ _ _] -> w5775
                          tunnel: "TEST STATION HAS REACHED 1 MILLION CYCLES, REPLACE  CONTROL RELAYS" -> [w5779 w5791 w5801 w5811 w5821 w5831 w5841 w5851 w5861 w5871]
                          tunnel: [_ w5790 _ _ _ _ _ _ _ _] -> w5773
                          tunnel: w5771 -> [_ w5789 _ _ _ _ _ _ _ _]
                          tunnel: [_ _ w5800 _ _ _ _ _ _ _] -> w5770
                          tunnel: w5769 -> [_ _ w5799 _ _ _ _ _ _ _]
                          tunnel: w5768 -> [_ _ _ w5810 _ _ _ _ _ _]
                          tunnel: [_ _ _ w5809 _ _ _ _ _ _] -> w5767
                          tunnel: w5766 -> [_ _ _ _ w5820 _ _ _ _ _]
                          tunnel: [_ _ _ _ w5819 _ _ _ _ _] -> w5765
                          tunnel: [_ _ _ _ _ w5830 _ _ _ _] -> w5764
                          tunnel: w5763 -> [_ _ _ _ _ w5829 _ _ _ _]
                          tunnel: w5762 -> [_ _ _ _ _ _ w5840 _ _ _]
                          tunnel: [_ _ _ _ _ _ w5839 _ _ _] -> w5761
                          tunnel: w5760 -> [_ _ _ _ _ _ _ w5850 _ _]
                          tunnel: [_ _ _ _ _ _ _ w5849 _ _] -> w5759
                          tunnel: w5758 -> [_ _ _ _ _ _ _ _ w5860 _]
                          tunnel: [_ _ _ _ _ _ _ _ w5859 _] -> w5757
                          tunnel: w5756 -> [_ _ _ _ _ _ _ _ _ w5870]
                          tunnel: [_ _ _ _ _ _ _ _ _ w5869] -> w5755
                          frame #0 {
                            n3178 = Greater?(x=w5780, y=w5783) -> (0:w5782:bool)
                            n3179 = case shown="True" w5782 {
                              tunnel: [w5784 0] -> w5781
                              tunnel: w5780 -> [w5784 _]
                              tunnel: w5779 -> [_ w5785]
                              frame False {
                              }
                              frame True {
                                n3180 = Concatenate Strings("LA01-1 ", w5785) -> (w5788:string)
                                n3181 = One Button Dialog(message=w5788) -> ()  [unwired: 1 in, 1 out]
                              }
                            }
                          }
                          frame #1 {
                            n3182 = Greater?(x=w5789, y=w5793) -> (0:w5792:bool)
                            n3183 = case shown="True" w5792 {
                              tunnel: [w5794 0] -> w5790
                              tunnel: w5789 -> [w5794 _]
                              tunnel: w5791 -> [_ w5795]
                              frame False {
                              }
                              frame True {
                                n3184 = Concatenate Strings("LA01-2 ", w5795) -> (w5798:string)
                                n3185 = One Button Dialog(message=w5798) -> ()  [unwired: 1 in, 1 out]
                              }
                            }
                          }
                          frame #2 {
                            n3186 = Greater?(x=w5799, y=w5803) -> (0:w5802:bool)
                            n3187 = case shown="True" w5802 {
                              tunnel: [w5804 0] -> w5800
                              tunnel: w5799 -> [w5804 _]
                              tunnel: w5801 -> [_ w5805]
                              frame False {
                              }
                              frame True {
                                n3188 = Concatenate Strings("LA02-1 ", w5805) -> (w5808:string)
                                n3189 = One Button Dialog(message=w5808) -> ()  [unwired: 1 in, 1 out]
                              }
                            }
                          }
                          frame #3 {
                            n3190 = Greater?(x=w5810, y=w5813) -> (0:w5812:bool)
                            n3191 = case shown="True" w5812 {
                              tunnel: [w5814 0] -> w5809
                              tunnel: w5810 -> [w5814 _]
                              tunnel: w5811 -> [_ w5815]
                              frame False {
                              }
                              frame True {
                                n3192 = Concatenate Strings("LA02-2 ", w5815) -> (w5818:string)
                                n3193 = One Button Dialog(message=w5818) -> ()  [unwired: 1 in, 1 out]
                              }
                            }
                          }
                          frame #4 {
                            n3194 = Greater?(x=w5820, y=w5823) -> (0:w5822:bool)
                            n3195 = case shown="True" w5822 {
                              tunnel: [w5824 0] -> w5819
                              tunnel: w5820 -> [w5824 _]
                              tunnel: w5821 -> [_ w5825]
                              frame False {
                              }
                              frame True {
                                n3196 = Concatenate Strings("LA03-1 ", w5825) -> (w5828:string)
                                n3197 = One Button Dialog(message=w5828) -> ()  [unwired: 1 in, 1 out]
                              }
                            }
                          }
                          frame #5 {
                            n3198 = Greater?(x=w5829, y=w5833) -> (0:w5832:bool)
                            n3199 = case shown="True" w5832 {
                              tunnel: [w5834 0] -> w5830
                              tunnel: w5829 -> [w5834 _]
                              tunnel: w5831 -> [_ w5835]
                              frame False {
                              }
                              frame True {
                                n3200 = Concatenate Strings("LA03-2 ", w5835) -> (w5838:string)
                                n3201 = One Button Dialog(message=w5838) -> ()  [unwired: 1 in, 1 out]
                              }
                            }
                          }
                          frame #6 {
                            n3202 = Greater?(x=w5840, y=w5843) -> (0:w5842:bool)
                            n3203 = case shown="True" w5842 {
                              tunnel: [w5844 0] -> w5839
                              tunnel: w5840 -> [w5844 _]
                              tunnel: w5841 -> [_ w5845]
                              frame False {
                              }
                              frame True {
                                n3204 = Concatenate Strings("LA04-1 ", w5845) -> (w5848:string)
                                n3205 = One Button Dialog(message=w5848) -> ()  [unwired: 1 in, 1 out]
                              }
                            }
                          }
                          frame #7 {
                            n3206 = Greater?(x=w5850, y=w5853) -> (0:w5852:bool)
                            n3207 = case shown="True" w5852 {
                              tunnel: [w5854 0] -> w5849
                              tunnel: w5850 -> [w5854 _]
                              tunnel: w5851 -> [_ w5855]
                              frame False {
                              }
                              frame True {
                                n3208 = Concatenate Strings("LA04-2 ", w5855) -> (w5858:string)
                                n3209 = One Button Dialog(message=w5858) -> ()  [unwired: 1 in, 1 out]
                              }
                            }
                          }
                          frame #8 {
                            n3210 = Greater?(x=w5860, y=w5863) -> (0:w5862:bool)
                            n3211 = case shown="True" w5862 {
                              tunnel: [w5864 0] -> w5859
                              tunnel: w5860 -> [w5864 _]
                              tunnel: w5861 -> [_ w5865]
                              frame False {
                              }
                              frame True {
                                n3212 = Concatenate Strings("LA05-1 ", w5865) -> (w5868:string)
                                n3213 = One Button Dialog(message=w5868) -> ()  [unwired: 1 in, 1 out]
                              }
                            }
                          }
                          frame #9 {
                            n3214 = Greater?(x=w5870, y=w5873) -> (0:w5872:bool)
                            n3215 = case shown="True" w5872 {
                              tunnel: [w5874 0] -> w5869
                              tunnel: w5870 -> [w5874 _]
                              tunnel: w5871 -> [_ w5875]
                              frame False {
                              }
                              frame True {
                                n3216 = Concatenate Strings("LA05-2 ", w5875) -> (w5878:string)
                                n3217 = One Button Dialog(message=w5878) -> ()  [unwired: 1 in, 1 out]
                              }
                            }
                          }
                        }
                        n3218 = Bundle By Name(cluster=w5777, "LAB01-1"=w5775, "LAB01-2"=w5773, "LAB02-1"=w5770, "LAB02-2"=w5767, "LAB03-1"=w5765, "LAB03-2"=w5764, "LAB04-1"=w5761, "LAB04-2"=w5759, "LAB05-1"=w5757, "LAB05-2"=w5755) -> (w5776:T9)
                        n3219 = local write "JIG RELAY CYCLES"(w5776) -> ()
                      }
                    }
                  }
                }
              }
            }
          }
          frame #21 {
            # "get temperature values"
            n3220 = local read "DAQ Simulate"() -> (w5891:bool)
            n3221 = local read "Temp Test Cal"() -> (w5888:dbl)
            n3222 = stacked-sequence {
              seq-local: [_ w5898 _] -> [_ _ w5945]
              tunnel: w5891 -> [_ _ w5958]
              tunnel: T15 {"1  (A) cal"=1.0, "1 (V) cal"=1.0, "1 (PF) cal"=1.0, "1 (TL) cal"=1.0, "1 (TN) cal"=1.0, "2 (A) cal"=1.0, "2 (V) cal"=1.0, "2 (PF) cal"=1.0, "2 (TL) cal"=1.0, "2 (TN) cal"=1.0} ("CAL LAB01") -> [_ _ w5957]
              tunnel: w5889 -> [_ _ w5956]
              tunnel: w5888 -> [_ _ w5955]
              tunnel: w5887 -> [_ _ w5954]
              tunnel: w5886 -> [_ _ w5953]
              tunnel: w5885 -> [_ _ w5952]
              tunnel: w5884 -> [_ _ w5951]
              tunnel: w5883 -> [_ _ w5950]
              tunnel: w5882 -> [_ _ w5949]
              tunnel: w5881 -> [_ _ w5948]
              tunnel: w5880 -> [_ _ w5947]
              tunnel: w5879 -> [_ _ w5946]
              frame #0 {
                n3223 = case shown="True" "Open Com Port" {
                  frame False {
                  }
                  frame True {
                    n3224 = local read "Select COM port"() -> (w5896:refnum<visa-resource-name>)
                    n3225 = call "sub vi-open serial port v1.vi"("Select COM port"=w5896) -> ("Error"=w5895:bool, "LOOPS"=w5894:i32, "VISA Com out"=w5893:refnum<visa-resource-name>)  [unwired: 12 in]
                    n3226 = local write "Com setup loops"(w5894) -> ()
                    n3227 = local write "Com Port Status"(w5895) -> ()
                    n3228 = local write "VISA Com out"(w5893) -> ()
                    n3229 = global write "Global 1.vi" "COM port"(w5893) -> ()
                  }
                }
              }
              frame #1 {
                # "only get temperature from initial valid temperature circuits, circuits detected at startup time"
                n3230 = local read "VISA Com out"() -> (w5906:refnum<visa-resource-name>)
                n3231 = global write "Global 1.vi" "COM port"(w5906) -> ()
                n3232 = local read "Temp read loop"() -> (w5903:dbl)
                n3233 = global write "Global 1.vi" "tmp dly lps"("Temp Delay Lps") -> ()
                n3234 = global write "Global 1.vi" "dly value"("Temp Value") -> ()
                n3235 = local read "jig cycle"() -> (w5907:dbl)
                n3236 = local read "on loops"() -> (w5909:dbl)
                n3237 = Equal?(x=w5903, y=1) -> (x = y?=w5900:bool)
                n3238 = Add(x=w5909, y=6) -> (x+y=w5910:dbl)
                n3239 = Equal?(x=w5907, y=w5910) -> (x = y?=w5901:bool)
                n3240 = And(x=w5901, y=w5900) -> (x .and. y?=w5899:bool)
                n3241 = Or(x=w5899, y="Read Temp") -> (x .or. y?=w5898:bool)
                n3242 = case shown="True" w5898 {
                  frame False {
                  }
                  frame True {
                    w5911 = TRUE
                    n3243 = local write "TEMP"(w5911) -> ()
                    n3244 = local write "Read Temp"(FALSE) -> ()
                    n3245 = stacked-sequence {
                      tunnel: 1.0 -> [_ _ _ _ w5944]
                      tunnel: "Temp Simulate" -> [_ _ _ _ w5943]
                      tunnel: w5911 -> [_ _ _ _ _]
                      frame #0 {
                        # "only switch relay on to reset temp circuits if busy testing"
                        n3246 = disable-structure shown="Enabled" {
                          frame Disabled {
                            n3247 = local read "Any Test Running"() -> ()  [unwired: 1 out]
                          }
                          frame Enabled {
                          }
                        }
                        n3248 = local read "USB OUT 0"() -> (w5916:bool[])
                        n3249 = local read "USB OUT 2"() -> (w5918:bool[])
                        n3250 = local read "USB OUT 1"() -> (w5917:bool[])
                        n3251 = Insert Into Array(array=w5918, index=7, new element=TRUE) -> (w5919:bool[])
                        n3252 = call "sub vi - Drive Relays All v6.vi"("Array #2"=w5919, "Array #1"=w5917, "Array #0"=w5916) -> ()  [unwired: 8 in, 1 out]
                      }
                      frame #1 {
                        # "time delay"
                        n3253 = Wait (ms)(milliseconds to wait=500) -> ()  [unwired: 1 out]
                      }
